vi "DetailedView.vi"(8 "error in (no error)":errorcluster, 10 "detailed":bool, 11 "TestView_Tree in":refnum<class "TestView_Base.lvclass">) -> (0 "error out":errorcluster, 3 "TestView_Tree out":refnum<class "TestView_Base.lvclass">)   [LabVIEW 2022 SP3, in "TestView_Base.lvlib" / "TestView_Base.lvclass"]
uses:
  TestView_Base.lvclass
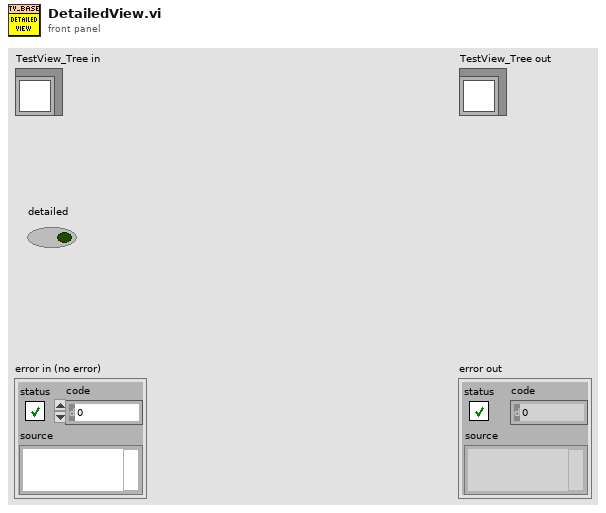
[diagram p1: front panel]
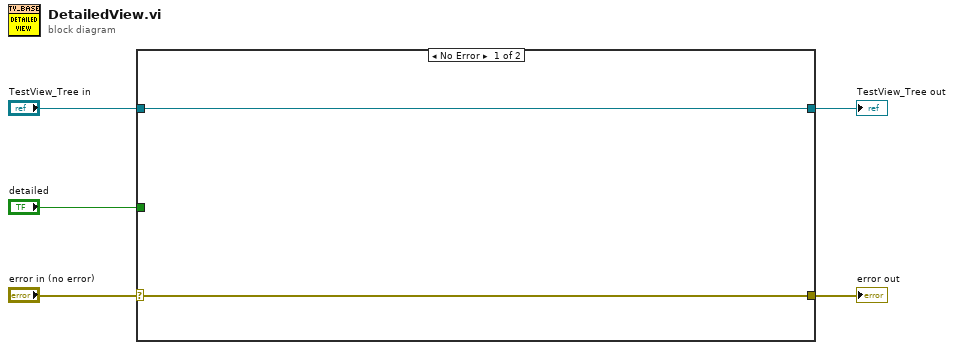
[diagram p0: block diagram]
diagram:
  n1 = case shown="No Error" "error in (no error)" {
    selector: "error in (no error)" -> [w7 w9]
    tunnel: [w7 w9] -> w4
    tunnel: [w6 w8] -> w2
    tunnel: "TestView_Tree in" -> [w6 w8]
    tunnel: "detailed" -> [_ _]
    frame No Error {
    }
    frame Error {
    }
  }
  "error out" <- w4
  "TestView_Tree out" <- w2
